vi "plot_txv.vi"(10 "txv":T1) -> (2 "XT":cluster{"time":dbl[], "velocity":dbl[]}[](array[cluster]))   [LabVIEW 2017, in "wf.lvlib"]
uses:
  wf.lvlib
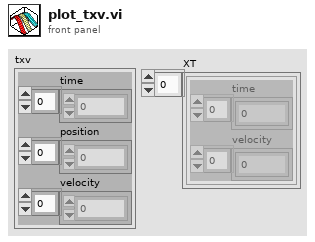
[diagram p1: front panel]
types:
  T1 = cluster{"time":dbl[], "position":dbl[], "velocity":dbl[]}
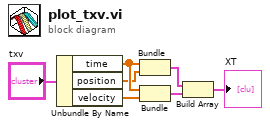
[diagram p0: block diagram]
diagram:
  n1 = Unbundle By Name("txv") -> ("time"=w7:dbl[], "position"=w6:dbl[], "velocity"=w5:dbl[])
  n2 = Bundle("time"=w7, "position"=w6) -> (w3:cluster{"time":dbl[], "position":dbl[]})  [unwired: 1 in]
  n3 = Bundle("time"=w7, "velocity"=w5) -> (w4:cluster{"time":dbl[], "velocity":dbl[]})  [unwired: 1 in]
  n4 = Build Array(w3, w4) -> (→"XT":cluster{"time":dbl[], "velocity":dbl[]}[])
